vi "Drive Controller.vi"(8 "error in":errorcluster) -> ()   [LabVIEW 2020]
doc: "This VI executes continuously carrying out the current operation and responding to updates or new operation requests. It will often contain the timing or control code that is difficult to place directly in TeleOp. This VI generally opens all sensors and motors and isolates the rest of the robot code from knowing implementation details of how the operations are carried out."
uses:
  <vilib>/Rock Robotics/WPI/Framework/Completion Status.ctl
  Drive Setpoints.ctl
  <vilib>/Rock Robotics/WPI/SafetyOutput/WPI_SafetyOutputConfigMenu.ctl
  <vilib>/Rock Robotics/WPI/RobotDrive/WPI_RobotDriveOpen2MotorWithVictorSPX.vi
panel:
  in  "Interactive Values":T1
  in  "Buttons":cluster{"Execute Cmd":bool, "Abort Cmd":bool}
  out "Command Timing":cluster{"Start Time (ms)":u32, "Iterations":i32}
  out "Status":T2
  out "Setpoints":T3(graph)
  out "Current\nCmd":string
  # "Tip: The graph shows the motor setpoints. It may also be helpful to observe inputs and sensor values.\nYou may also want to display tuning or debugging controls."
  # "Interactive Command: You may fill in the settings for a command\nand schedule it with the Execute button. You can observe and abort\nany command while fine tuning the code for the controller."
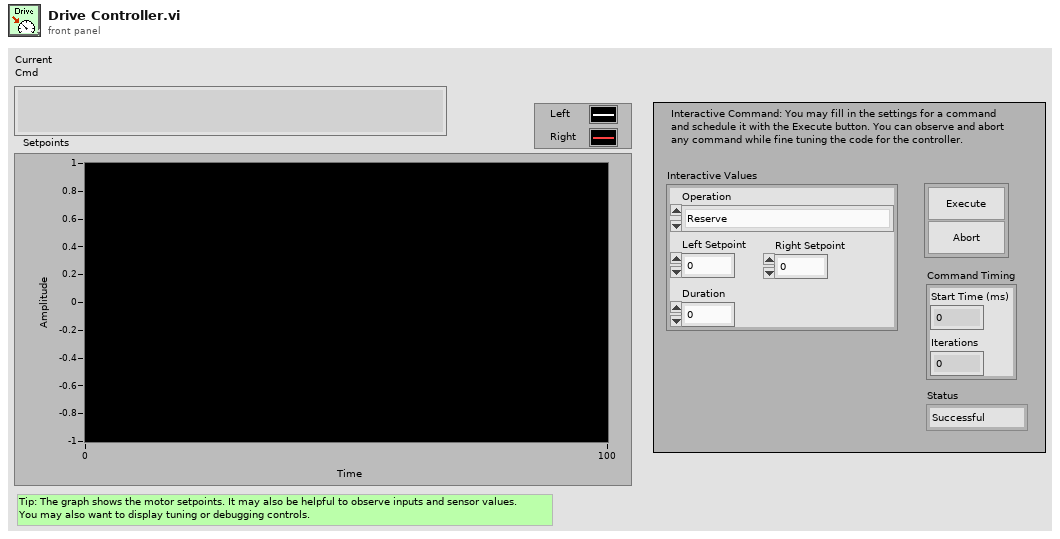
[diagram p1: front panel]
types:
  T1 = typedef "Drive Setpoints.ctl" = cluster{"Operation":enum16{"Reserve", "Read Current", "Immediate", "Drive for Time", "Drive for Distance"}, "Left Setpoint":dbl, "Right Setpoint":dbl, "Duration":dbl}
  T2 = typedef "Completion Status.ctl" = enum16{"Successful", "Aborted", "Incomplete"}
  T3 = cluster{"Left Setpoint":dbl, "Right Setpoint":dbl}
  T4 = typedef "WPI_SafetyOutputConfigMenu.ctl" = enum16{"Enable", "Disable"}
  T5 = typedef "WPI_RobotDriveDevRef.ctl" = cluster{"DevStatus":errorcluster, "Motors[]":T6[], "Square Inputs":bool, "Max Output":dbl}
  T6 = typedef "WPI_MotorControlDeviceRef.ctl" = cluster{"DeviceStatus":errorcluster, "Type":T7, "PWM":cluster{"PWM Channel":T8, "DeadBand":T9}, "CAN":cluster{"Device Number":u8, "SetOutput VI Ref":variant, "GetOutput VI Ref":variant, "Enable VI Ref":variant, "Disable VI Ref":variant, "Data":variant}, "Invert":bool, "DIO PWM":cluster{"PWM \"Enable\" Channel":T8, "DIOChannel":T10, "PWM Rate":dbl}}
  T7 = typedef "WPI_MotorControlType.ctl" = enum16{"PWM", "CAN", "DIO PWM"}
  T8 = typedef "FPGA_DIOPWMChannel.ctl" = enum8{"PWM 0", "PWM 1", "PWM 2", "PWM 3", "PWM 4", "PWM 5", "PWM 6", "PWM 7", "PWM 8", "PWM 9", "PWM MXP 0", "PWM MXP 1", "PWM MXP 2", "PWM MXP 3", "PWM MXP 4", "PWM MXP 5", "PWM MXP 6", "PWM MXP 7", "PWM MXP 8", "PWM MXP 9", "Invalid"}
  T9 = typedef "WPI_PWMDeadband.ctl" = cluster{"Name":string, "maxPositivePwm":i32, "minPositivePwm":i32, "centerPwm":i32, "maxNegativePwm":i32, "minNegativePwm":i32, "angularRange":u16}
  T10 = typedef "FPGA_DIOChannel.ctl" = enum8{"DIO 0", "DIO 1", "DIO 2", "DIO 3", "DIO 4", "DIO 5", "DIO 6", "DIO 7", "DIO 8", "DIO 9", "DIO MXP 0", "DIO MXP 1", "DIO MXP 2", "DIO MXP 3", "DIO MXP 4", "DIO MXP 5", "DIO MXP 6", "DIO MXP 7", "DIO MXP 8", "DIO MXP 9", "DIO MXP 10", "DIO MXP 11", "DIO MXP 12", "DIO MXP 13", "DIO MXP 14", "DIO MXP 15", "SPI Port CS1", "SPI Port CS2", "SPI Port CS3", "SPI Port MISO", "SPI Port MOSI", "Invalid"}
  T11 = typedef "Command Status Info.ctl" = cluster{"Name":string, "Status":T2, "notifier out":T12}
  T12 = typedef "Completion Notifier.ctl" = refnum<notifier>
  T13 = cluster{"SubSystem Data":T1, cluster{"Start Time (ms)":u32, "Iterations":i32}, cluster{"Command Info":T11, "Description":string, "Default Command":T1, "queue out":refnum<queue>, "Subsystem Name":string}}
  T14 = enum16{"Reserve", "Read Current", "Immediate", "Drive for Time", "Drive for Distance"}
  T15 = cluster{"SubSystem Data":T1, cluster{"Start Time (ms)":u32, "Iterations":i32}, "Default Command Arguments":cluster{"Command Info":T11, "Description":string, "Default Command":T1, "queue out":refnum<queue>, "Subsystem Name":string}}
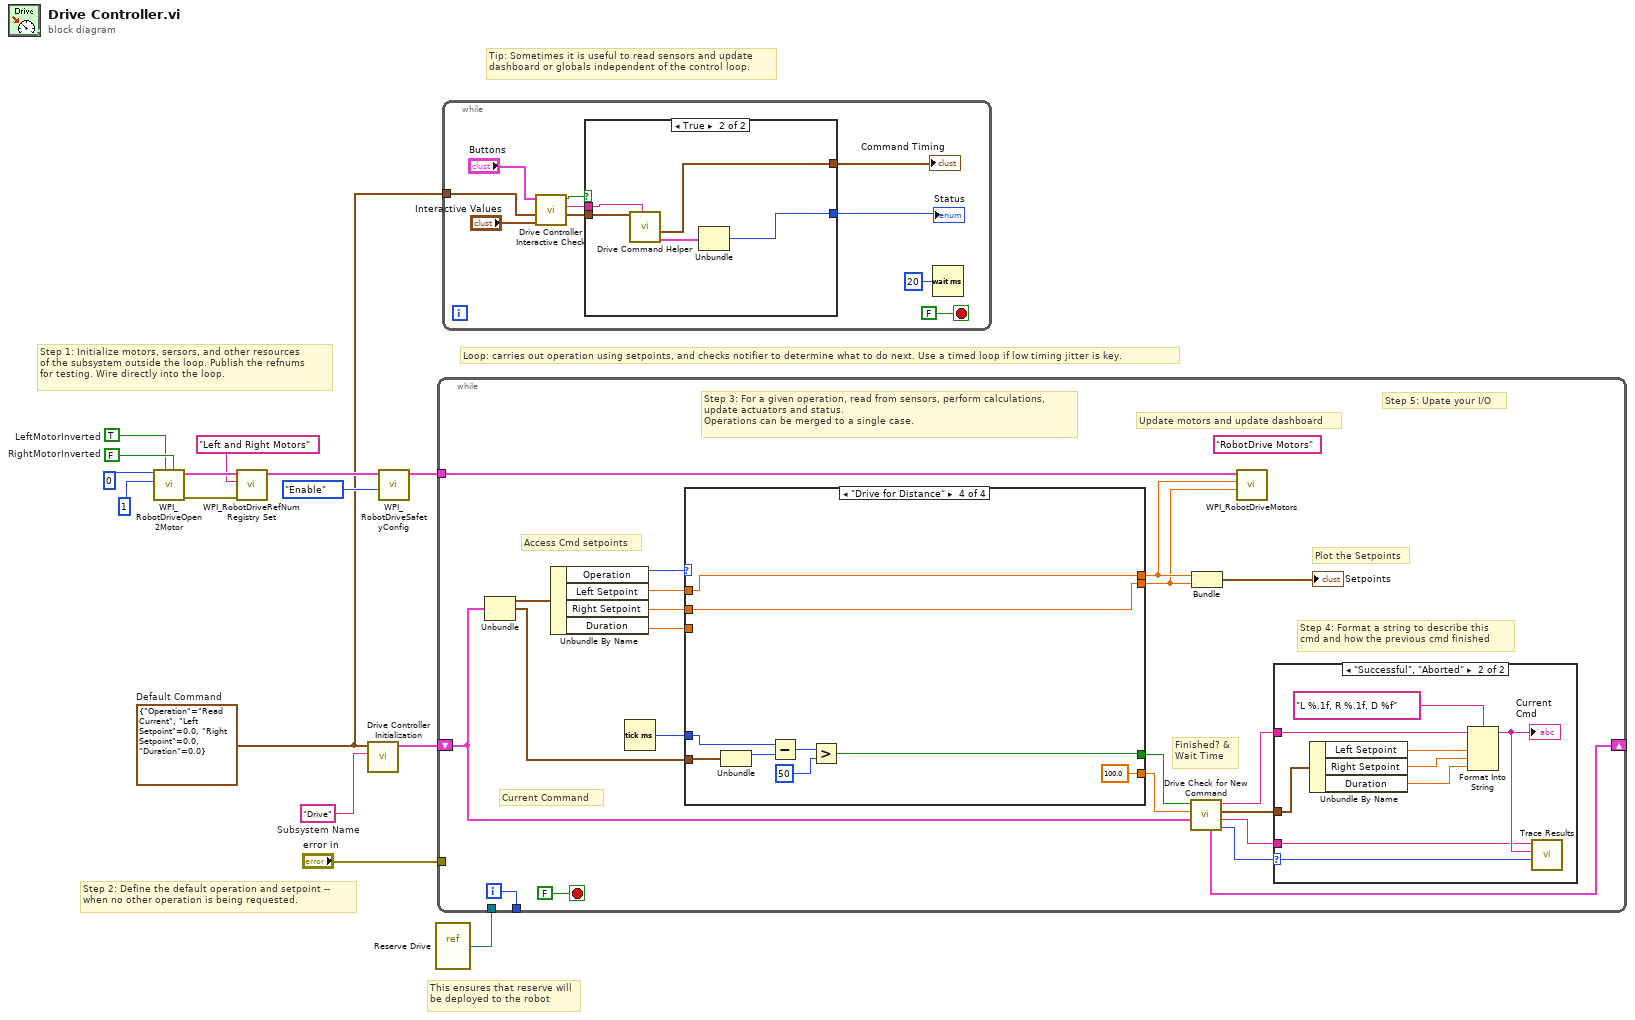
[diagram p0: block diagram]
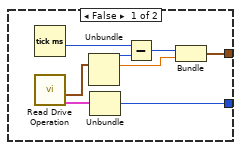
[diagram p2: hidden frame]
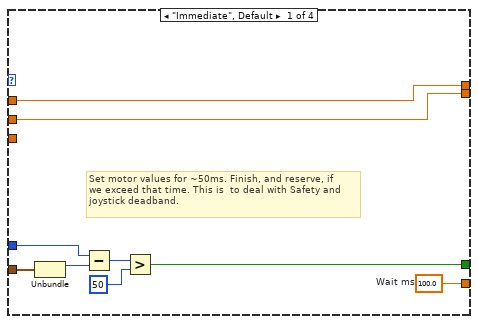
[diagram p4: hidden frame]
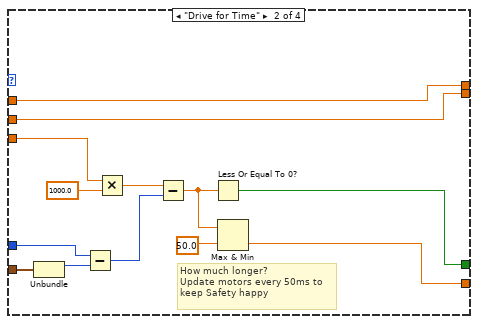
[diagram p5: hidden frame]
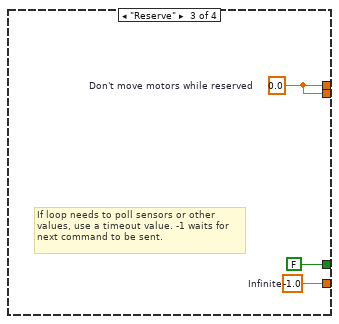
[diagram p6: hidden frame]
diagram:
  w11 = TRUE  # LeftMotorInverted
  w12 = FALSE  # RightMotorInverted
  w1 = T1 {"Operation"=enum."Read Current", "Left Setpoint"=0.0, "Right Setpoint"=0.0, "Duration"=0.0}  # Default Command
  w15 = "Drive"  # Subsystem Name
  # "This ensures that reserve will\nbe deployed to the robot"
  # "Tip: Sometimes it is useful to read sensors and update\ndashboard or globals independent of the control loop."
  # "Step 2: Define the default operation and setpoint --\nwhen no other operation is being requested."
  # "Step 1: Initialize motors, sersors, and other resources\nof the subsystem outside the loop. Publish the refnums\nfor testing. Wire directly into the loop."
  # "Loop: carries out operation using setpoints, and checks notifier to determine what to do next. Use a timed loop if low timing jitter is key."
  n1 = call-poly <vilib>:"WPI_RobotDriveOpen2Motor.vi"("Right Motor Inverted"=w12, "Left Motor Inverted"=w11, "Right Motor"=u8 1 ("Left Motor"), "Left Motor"=u8 0) -> ("error out"=w8:errorcluster, "RobotDriveDevRef"=w10:T5)  [unwired: 1 in, 5 out]
  n2 = call <vilib>:"WPI_RobotDriveRefNum Registry Set.vi"("error in (no error)"=w8, "refnum name"="Left and Right Motors", "RobotDriveDevRef"=w10) -> ("RobotDriveDevRef"=w7:T5)  [unwired: 1 in, 7 out]
  n3 = call "Drive Controller Initialization.vi"("Subsystem Name"=w15, "Default Command"=w1) -> ("Current Command"=w3:T13)  [unwired: 9 in]
  n4 = call <vilib>:"WPI_RobotDriveSafetyConfig.vi"("mode"=WPI_SafetyOutputConfigMenu."Enable", "RobotDriveDevRef"=w7) -> ("RobotDriveDevRef"=w5:T5)  [unwired: 8 in, 1 out]
  n5 = vi-ref "Reserve Drive.vi"() -> (w2:refnum<vi>)
  n6 = while {
    shift-right: [w23] -> _
    shift-left: w3 -> [w16]
    tunnel: [w35] -> _
    tunnel: w5 -> [w31]
    tunnel: "error in" -> [_]
    tunnel: w2 -> [_]
    i -> [w35]
    stop <- FALSE stop-if-true
    (unwired) "RobotDrive Motors" ("Name")
    # "Step 5: Upate your I/O"
    # "Step 4: Format a string to describe this\ncmd and how the previous cmd finished"
    # "Current Command"
    # "Update motors and update dashboard"
    # "Plot the Setpoints"
    # "Access Cmd setpoints"
    # "Finished? &\nWait Time"
    # "Step 3: For a given operation, read from sensors, perform calculations,\nupdate actuators and status.\nOperations can be merged to a single case."
    n7 = Unbundle(w16) -> ("SubSystem Data"=w30:T1, w17:cluster{"Start Time (ms)":u32, "Iterations":i32})  [unwired: 1 out]
    n8 = Unbundle By Name(w30) -> ("Operation"=w29:T14, "Left Setpoint"=w28:dbl, "Right Setpoint"=w27:dbl, "Duration"=w26:dbl)
    n9 = Tick Count (ms)() -> (millisecond timer value=w25:u32)
    n10 = case shown="\"Drive for Distance\"" w29 {
      tunnel: [w54 w55 w70 100.0 ("Infinite")] -> w22
      tunnel: [w47 w62 FALSE ("ignore previous (F)") w74] -> w21
      tunnel: w17 -> [w46 w64 _ w75]
      tunnel: [w53 w61 w68 w72] -> w33
      tunnel: [w52 w60 w68 w71] -> w32
      tunnel: w28 -> [w53 w61 _ w72]
      tunnel: w27 -> [w52 w60 _ w71]
      tunnel: w26 -> [_ w59 _ _]
      tunnel: w25 -> [w48 w58 _ w76]
      frame "Immediate", Default {
        w54 = 100.0  # Wait ms
        # "Set motor values for ~50ms. Finish, and reserve, if\nwe exceed that time. This is  to deal with Safety and\njoystick deadband."
        n11 = Unbundle(w46) -> ("Start Time (ms)"=w49:u32)  [unwired: 1 out]
        n12 = Subtract(x=w48, y=w49) -> (x-y=w50:u32)
        n13 = Greater?(x=w50, y=u8 50 ("Left Motor")) -> (0:w47:bool)
      }
      frame "Drive for Time" {
        # "How much longer?\nUpdate motors every 50ms to\nkeep Safety happy"
        n14 = Unbundle(w64) -> ("Start Time (ms)"=w63:u32)  [unwired: 1 out]
        n15 = Subtract(x=w58, y=w63) -> (x-y=w67:u32)
        n16 = Multiply(x=w59, y=1000.0) -> (x*y=w66:dbl)
        n17 = Subtract(x=w66, y=w67) -> (x-y=w57:dbl)
        n18 = Less Or Equal To 0?(x=w57) -> (x <= 0?=w62:bool)
        n19 = Max & Min(x=w57, y=50.0) -> (min(x,y)=w55:dbl)  [unwired: 1 out]
      }
      frame "Reserve" {
        w68 = 0.0  # Don't move motors while reserved
        w70 = -1.0  # Infinite
        # "If loop needs to poll sensors or other\nvalues, use a timeout value. -1 waits for\nnext command to be sent."
      }
      frame "Drive for Distance" {
        n20 = Unbundle(w75) -> ("Start Time (ms)"=w79:u32)  [unwired: 1 out]
        n21 = Subtract(x=w76, y=w79) -> (x-y=w78:u32)
        n22 = Greater?(x=w78, y=u8 50 ("Left Motor")) -> (0:w74:bool)
      }
    }
    n23 = call "Drive Check for New Command.vi"("input cluster"=w16, "Wait time (ms)"=w22, "Finished?"=w21) -> ("Completion"=w24:T2, "Subsystem Name"=w18:string, "Current Command"=w19:T1, "Initial Trace String"=w20:string, "Next Command"=w23:T15)  [unwired: 4 in]
    n24 = Bundle("Left Setpoint"=w33, "Right Setpoint"=w32) -> (→"Setpoints":T3)  [unwired: 1 in]
    n25 = call <vilib>:"WPI_RobotDriveMotors.vi"("RightSpeed"=w32, "LeftSpeed"=w33, "RobotDriveDevRef"=w31) -> ()  [unwired: 1 in, 8 out]
    n26 = case shown="\"Successful\", \"Aborted\"" w24 {
      selector: w24 -> [_ w45]
      tunnel: w20 -> [_ w40]
      tunnel: w19 -> [_ w41]
      tunnel: w18 -> [_ w37]
      frame "Incomplete", Default {
        # "Continuing current command"
      }
      frame "Successful", "Aborted" {
        # "Report and setup for next command"
        n27 = Unbundle By Name(w41) -> ("Left Setpoint"=w43:dbl, "Right Setpoint"=w44:dbl, "Duration"=w38:dbl)
        n28 = Format Into String(format string="L %.1f, R %.1f, D %f", initial string=w40, w43, w44, w38) -> (resulting string=w39:string)  [unwired: 1 in, 1 out]
        "Current\nCmd" <- w39
        n29 = call <vilib>:"Trace Results.vi"("Status of previous command"=w45, "Description"=w39, "Subsystem"=w37) -> ()  [unwired: 9 in]
      }
    }
  }
  n30 = while {
    tunnel: w1 -> [w81]
    stop <- FALSE stop-if-true
    n31 = call "Drive Controller Interactive Check.vi"("Interactive Command In"="Interactive Values", "Default Command"=w81, "Buttons"="Buttons") -> ("Interactive Command Out"=w83:T1, "Trace String"=w84:string, "Schedule"=w85:bool)  [unwired: 6 in]
    n32 = case shown="True" w85 {
      tunnel: [w94 w102] -> w86
      tunnel: [w93 w98] -> w87
      tunnel: w84 -> [_ w100]
      tunnel: w83 -> [_ w99]
      frame False {
        n33 = Tick Count (ms)() -> (millisecond timer value=w97:u32)
        n34 = call "Read Drive Operation.vi"() -> ("Command Info"=w91:T11, "SubSystem Data"=w90:T1)  [unwired: 9 in, 1 out]
        n35 = Unbundle(w90) -> ("Operation"=w95:T14, "Left Setpoint"=w92:dbl)  [unwired: 2 out]
        n36 = Unbundle(w91) -> ("Status"=w94:T2)  [unwired: 2 out]
        n37 = Subtract(x=w97, y=w95) -> (x-y=w96:u32)
        n38 = Bundle(w96, "Left Setpoint"=w92) -> (w93:cluster{u32, "Left Setpoint":dbl})  [unwired: 1 in]
      }
      frame True {
        n39 = call "Drive Command Helper.vi"("Description"=w100, "SubSystem Data"=w99) -> ("Command Info Out"=w101:T11, "Command Timing"=w98:cluster{"Start Time (ms)":u32, "Iterations":i32})  [unwired: 7 in, 1 out]
        n40 = Unbundle(w101) -> ("Status"=w102:T2)  [unwired: 2 out]
      }
    }
    "Status" <- w86
    "Command Timing" <- w87
    n41 = Wait (ms)(milliseconds to wait=u32 20) -> ()  [unwired: 1 out]
  }
